vi "complimentaryFilter.vi"(4 "alpha":dbl=0.99 format="%#_13g", 10 "low pass component":dbl, 11 "high pass component":dbl) -> (3 "filtered signal":dbl)   [LabVIEW 2020]
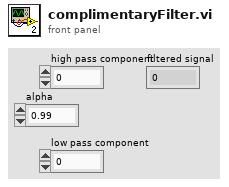
[diagram p1: front panel]
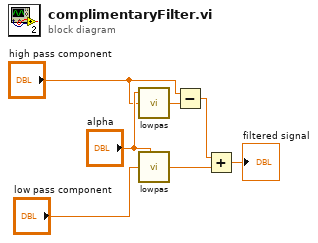
[diagram p0: block diagram]
diagram:
  n1 = call "lowpas.vi"("alpha"="alpha", "x"="high pass component") -> ("Numeric"=w2:dbl)  [unwired: 5 in]
  n2 = call "lowpas.vi"("alpha"="alpha", "x"="low pass component") -> ("Numeric"=w5:dbl)  [unwired: 5 in]
  n3 = Subtract(x="high pass component", y=w2) -> (x-y=w4:dbl)
  n4 = Add(x=w4, y=w5) -> (x+y=→"filtered signal":dbl)
